vi "DataReader.vi"() -> ()   [LabVIEW 2016]
uses:
  <vilib>/express/express shared/transition.llb/Dynamic To Waveform Array.vi
  <vilib>/express/express signal manip/GetorSetDDTAttributes/Get DDT Attributes/Get DDT Properties.xnode
panel:
  out "Time Span":dbl
  in  "Liquid Type":bool
  in  "Gas Type":bool
  in  "Move Back":bool
  in  "Advance":bool
  in  "End Time":dbl
  in  "Start Time":dbl
  in  "Refresh Button":bool
  out "TCp-2O-3O":dynamicdata(graph)
  out "TCp-2P-3P":dynamicdata(graph)
  out "TCp-1F-2F":dynamicdata(graph)
  out "PT-2P-3P":dynamicdata(graph)
  out "PT-1E-2E":dynamicdata(graph)
  out "PT-1F-2F-3F":dynamicdata(graph)
  out "PT-2O-3O":dynamicdata(graph)
  out "LC-1E":dynamicdata(graph)
  out "TCp-3P":dynamicdata(graph)
  out "TCp-2P":dynamicdata(graph)
  out "TCp-1P":dynamicdata(graph)
  out "TCp-2F":dynamicdata(graph)
  out "TCp-1F":dynamicdata(graph)
  out "TCp-3O":dynamicdata(graph)
  out "TCp-2O":dynamicdata(graph)
  out "TCp-1O":dynamicdata(graph)
  out "FM-F":dynamicdata(graph)
  out "FM-O":dynamicdata(graph)
  out "PT-3P":dynamicdata(graph)
  out "PT-2P":dynamicdata(graph)
  out "PT-1P":dynamicdata(graph)
  out "PT-L":dynamicdata(graph)
  out "PT-2E":dynamicdata(graph)
  out "PT-1E":dynamicdata(graph)
  out "PT-TI":dynamicdata(graph)
  out "PT-IF":dynamicdata(graph)
  out "PT-IO":dynamicdata(graph)
  out "PT-3F":dynamicdata(graph)
  out "PT-2F":dynamicdata(graph)
  out "PT-1F":dynamicdata(graph)
  out "PT-3O":dynamicdata(graph)
  out "PT-2O":dynamicdata(graph)
  out "PT-1O":dynamicdata(graph)
  # "Water"
  # "N2"
  # "Kerosene"
  # "O2"
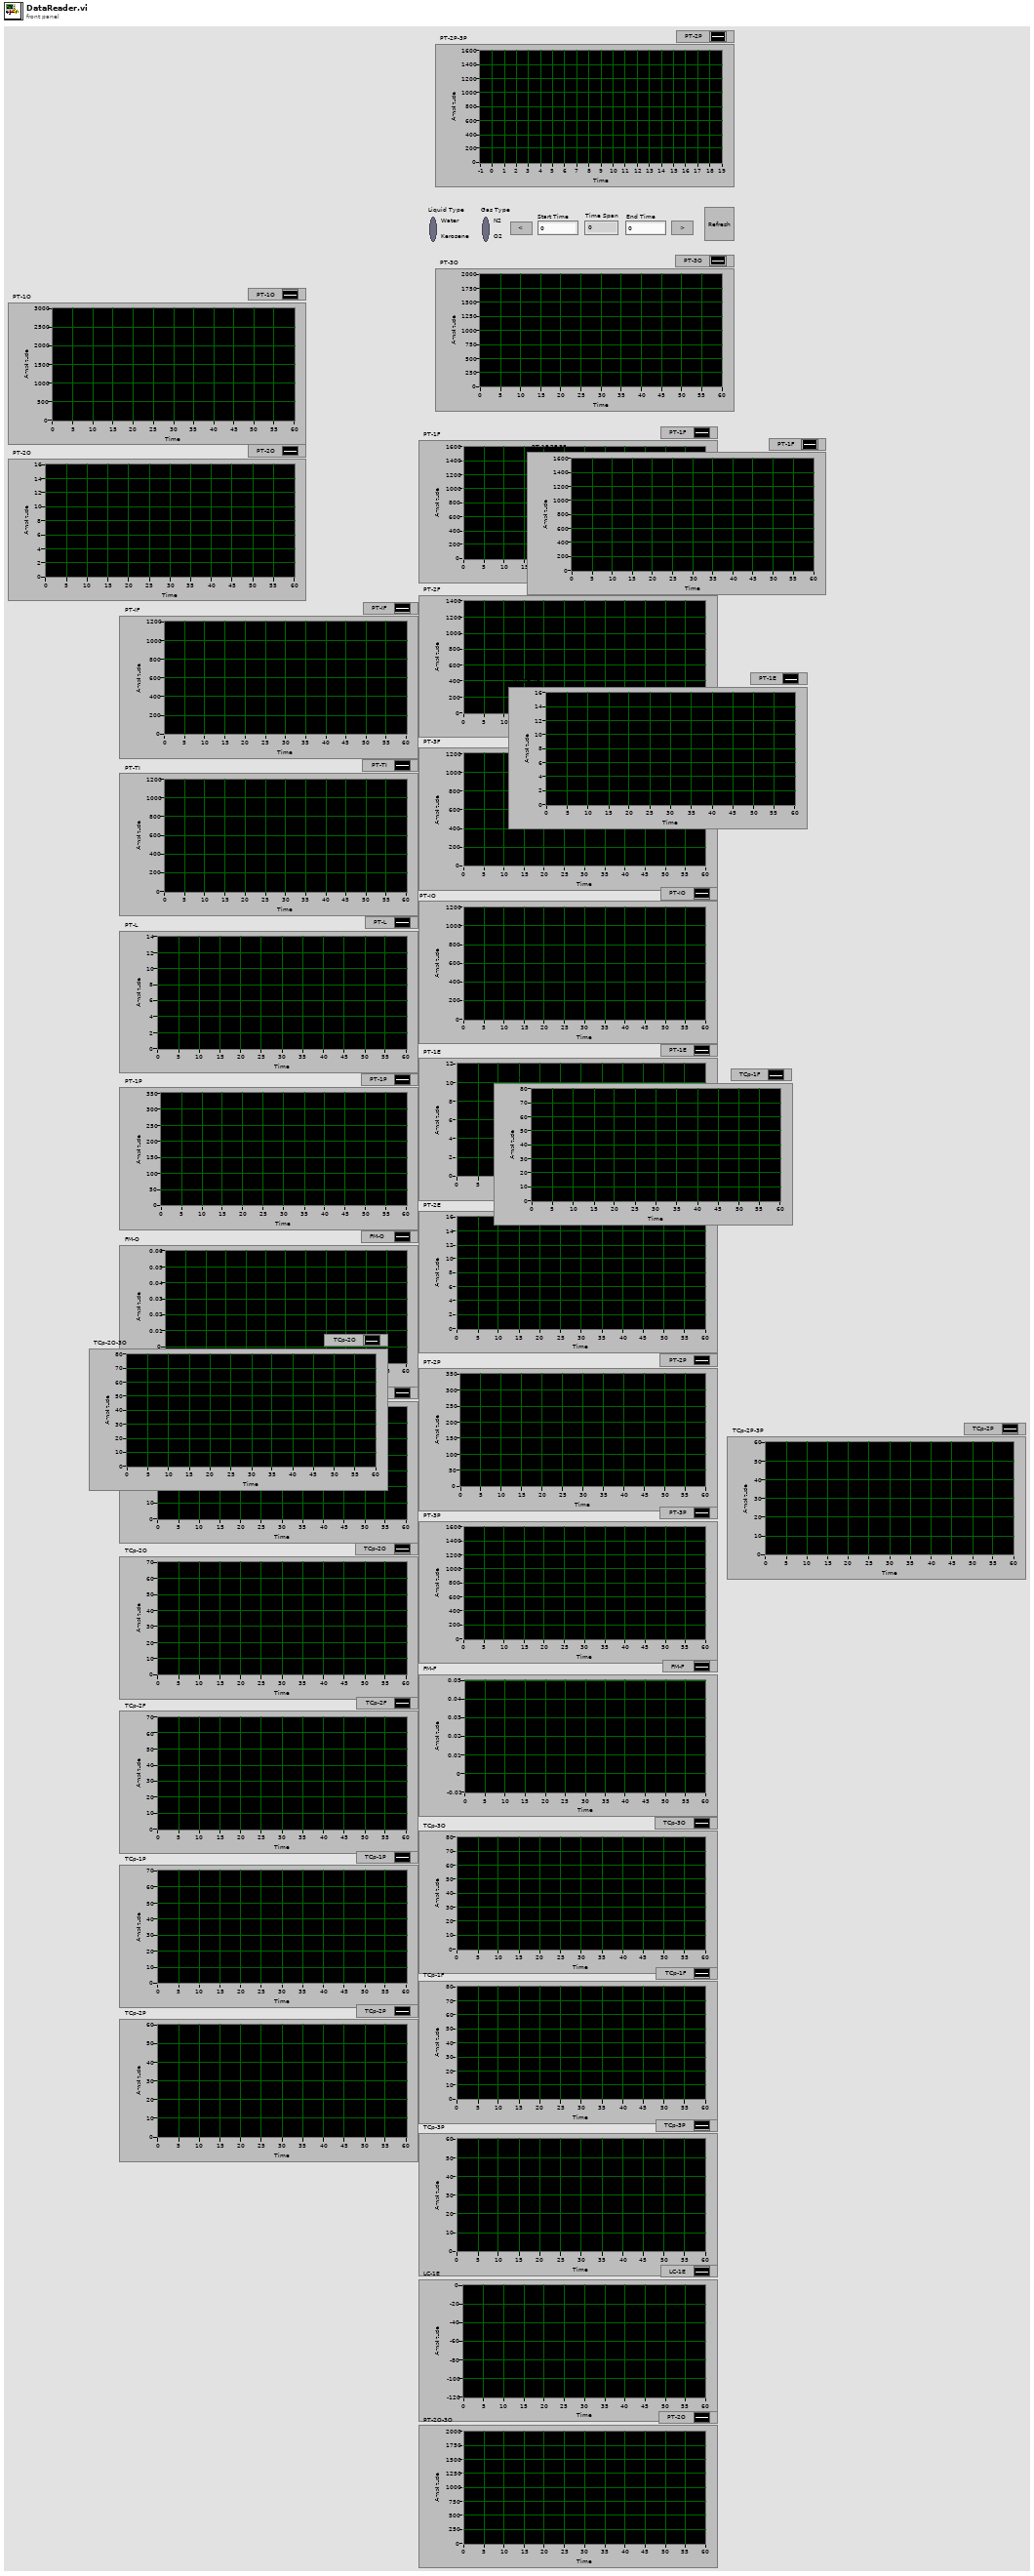
[diagram p1: front panel]
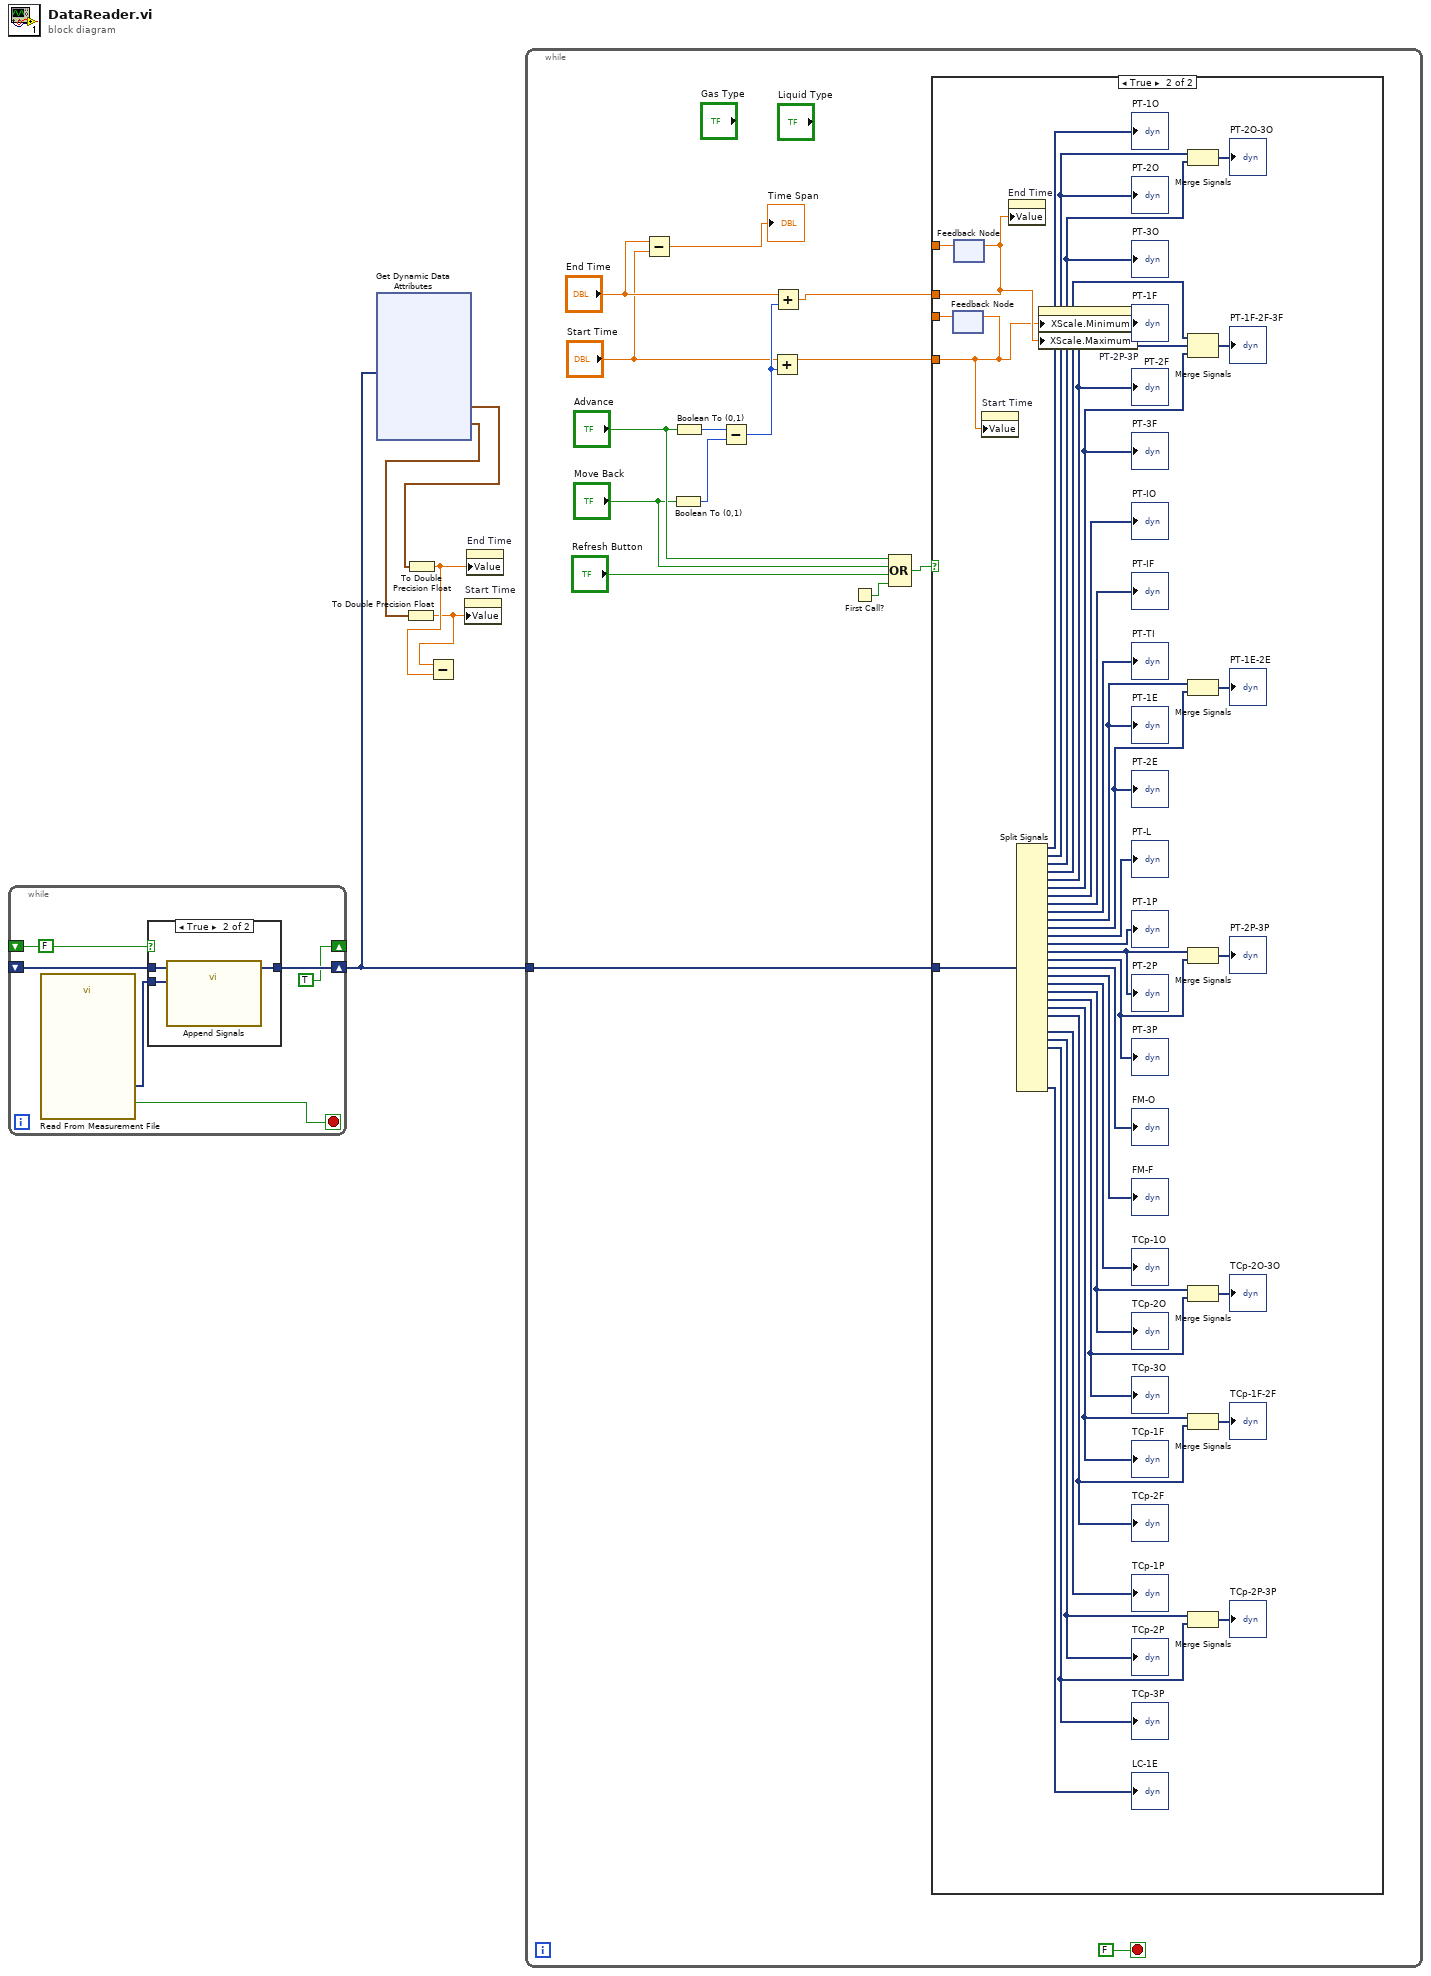
[diagram p0: block diagram]
diagram:
  n1 = while {
    shift-right: [w10] -> w5
    shift-left: _ -> [w11]
    shift-right: [TRUE] -> _
    shift-left: FALSE -> [w7]
    stop <- w12 stop-if-true
    n2 = call "Read From Measurement File"() -> ("Signals"=w9:dynamicdata, "EOF?"=w12:bool)  [unwired: 6 in, 4 out]
    n3 = case shown="True" w7 {
      tunnel: w11 -> [_ w16]
      tunnel: [w13 w15] -> w10
      tunnel: w9 -> [w13 w14]
      frame False {
      }
      frame True {
        n4 = call "Append Signals"("Input Signal B"=w14, "Input Signal A"=w16) -> ("Appended Signals"=w15:dynamicdata)  [unwired: 8 in, 1 out]
      }
    }
  }
  n5 = xnode "Get Dynamic Data Attributes"("Signals In"=w5) -> ("Timestamp"=w3:timestamp, "Start Timestamp"=w4:timestamp)  [unwired: 2 in, 2 out]
  n6 = To Double Precision Float(number=w4) -> (double precision float=w1:dbl)
  n7 = To Double Precision Float(number=w3) -> (double precision float=w2:dbl)
  n8 = Subtract(x=w1, y=w2) -> ()  [unwired: 1 out]
  n9 = property on="Start Time" class="DigNum (strict)"("Value"=w1) -> ()  [unwired: 2 in, 2 out]
  n10 = property on="End Time" class="DigNum (strict)"("Value"=w2) -> ()  [unwired: 2 in, 2 out]
  n11 = while {
    tunnel: w5 -> [w28]
    stop <- FALSE stop-if-true
    n12 = Subtract(x="End Time", y="Start Time") -> (x-y=→"Time Span":dbl)
    n13 = Boolean To (0,1)(Boolean="Move Back") -> (0, 1=w24:i16)
    n14 = Boolean To (0,1)(Boolean="Advance") -> (0, 1=w25:i16)
    n15 = Subtract(x=w25, y=w24) -> (x-y=w22:i16)
    n16 = Add(x="Start Time", y=w22) -> (x+y=w23:dbl)
    n17 = Add(x="End Time", y=w22) -> (x+y=w19:dbl)
    n18 = First Call?() -> (First Call?: T/F=w17:bool)
    n19 = Compound Arithmetic op=OR("Advance", "Move Back", "Refresh Button", w17) -> (w29:bool)
    n20 = case shown="True" w29 {
      tunnel: w28 -> [_ w71]
      tunnel: w19 -> [w33 w35]
      tunnel: w23 -> [w32 w34]
      tunnel: [w33 w37] -> _
      tunnel: [w32 w36] -> _
      frame False {
      }
      frame True {
        n21 = feedback-in #1(w34) -> ()
        n22 = feedback #1() -> (w36:dbl)  [unwired: 1 in]
        n23 = feedback #2() -> (w37:dbl)  [unwired: 1 in]
        n24 = feedback-in #2(w35) -> ()
        n25 = property on="Start Time" class="DigNum (strict)"("Value"=w34) -> ()  [unwired: 2 in, 2 out]
        n26 = property on="End Time" class="DigNum (strict)"("Value"=w35) -> ()  [unwired: 2 in, 2 out]
        n27 = Split Signals(w71) -> (→"PT-1O":dynamicdata, w58:dynamicdata, w59:dynamicdata, w56:dynamicdata, w55:dynamicdata, w54:dynamicdata, →"PT-IO":dynamicdata, →"PT-IF":dynamicdata, →"PT-TI":dynamicdata, w52:dynamicdata, w51:dynamicdata, →"PT-L":dynamicdata, →"PT-1P":dynamicdata, w49:dynamicdata, w48:dynamicdata, →"FM-O":dynamicdata, →"FM-F":dynamicdata, →"TCp-1O":dynamicdata, w39:dynamicdata, w38:dynamicdata, w46:dynamicdata, w45:dynamicdata, →"TCp-1P":dynamicdata, w43:dynamicdata, w42:dynamicdata, →"LC-1E":dynamicdata)  [unwired: 31 in, 5 out]
        "PT-2O" <- w58
        "PT-3O" <- w59
        "PT-1F" <- w56
        "PT-2F" <- w55
        "PT-3F" <- w54
        "PT-1E" <- w52
        "PT-2E" <- w51
        "PT-2P" <- w49
        "PT-3P" <- w48
        "TCp-2O" <- w39
        "TCp-3O" <- w38
        "TCp-1F" <- w46
        "TCp-2F" <- w45
        "TCp-2P" <- w43
        "TCp-3P" <- w42
        n28 = property on="PT-2P-3P" class="WFGraph (strict)"("XScale.Minimum"=w34, "XScale.Maximum"=w35) -> ()  [unwired: 2 in, 2 out]
        n29 = Merge Signals(w58, w59) -> (→"PT-2O-3O":dynamicdata)
        n30 = Merge Signals(w56, w55, w54) -> (→"PT-1F-2F-3F":dynamicdata)
        n31 = Merge Signals(w52, w51) -> (→"PT-1E-2E":dynamicdata)
        n32 = Merge Signals(w49, w48) -> (→"PT-2P-3P":dynamicdata)
        n33 = Merge Signals(w39, w38) -> (→"TCp-2O-3O":dynamicdata)
        n34 = Merge Signals(w46, w45) -> (→"TCp-1F-2F":dynamicdata)
        n35 = Merge Signals(w43, w42) -> (→"TCp-2P-3P":dynamicdata)
      }
    }
  }
